vi "Main_SelectROI_on_ExtDispl.vi"() -> ()   [LabVIEW 2020]
panel:
  out "ROI Descriptor":T1 {"Contours"."Type" items=["No Selection", "Point", "Line", "Rectangle", "Oval", "Polygon", "Freehand Region", "Annulus", "Unused2", "Unused3", "Broken Line", "Freehand Line", "Rotated Rectangle"]}
  in  "Event Button":bool
  out "Image":T2(plugin-control)
  out "error OUT":errorcluster
  in  "stop":bool
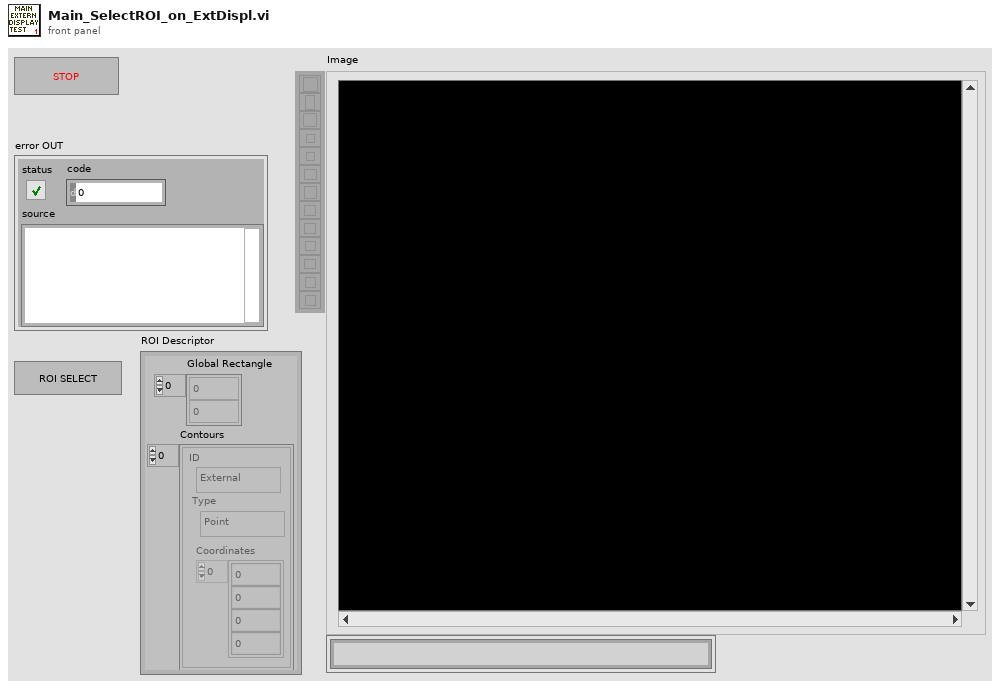
[diagram p1: front panel]
types:
  T1 = typedef "ROI Descriptor" = cluster{"Global Rectangle":i32[], "Contours":cluster{"ID":enum32{"External", "Internal"}, "Type":u32, "Coordinates":i32[]}[]}
  T2 = typedef "IMAQ Image.ctl" = refnum<image>
  T3 = typedef "Image Type" = u32
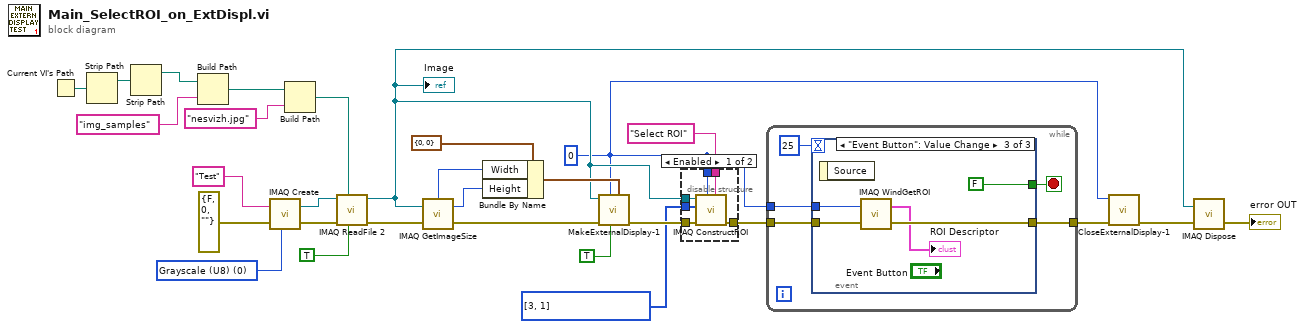
[diagram p0: block diagram]
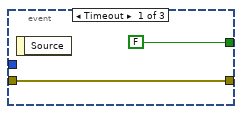
[diagram p3: hidden frame]
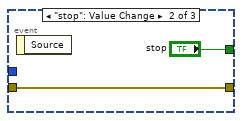
[diagram p4: hidden frame]
diagram:
  w9 = u32[] [3, 1] items=["No Selection", "Point", "Line", "Rectangle", "Oval", "Polygon", "Freehand Region", "Annulus", "Zoom", "Pan", "Broken Line", "Freehand Line", "Rotated Rectangle"] ("Tools")
  w8 = 0
  w27 = T3 0 items=["Grayscale (U8)", "Grayscale (I16)", "Grayscale (SGL)", "Complex (CSG)", "RGB (U32)", "HSL (U32)", "RGB (U64)", "Grayscale (U16)"] ("Image Type")
  n1 = Current VI's Path() -> (path=w4:path)
  n2 = Strip Path(path=w4) -> (stripped path=w3:path)  [unwired: 1 out]
  n3 = Strip Path(path=w3) -> (stripped path=w2:path)  [unwired: 1 out]
  n4 = Build Path(base path=w2, name or relative path="img_samples") -> (appended path=w5:path)
  n5 = call "IMAQ Create"("Image Name"="Test", "Image Type"=w27, "error in (no error)"=errorcluster {"status"=FALSE, "code"=0, "source"=""}) -> ("New Image"=w25:T2, "error out"=w26:errorcluster)  [unwired: 2 in]
  n6 = Build Path(base path=w5, name or relative path="nesvizh.jpg") -> (appended path=w1:path)
  n7 = call "IMAQ ReadFile 2"("Use File Path Image Type"=TRUE, "File Path"=w1, "error in (no error)"=w26, "Image"=w25) -> ("error out"=w21:errorcluster, "Image Out"=w11:T2)  [unwired: 3 in, 3 out]
  "Image" <- w11
  n8 = call "IMAQ GetImageSize"("Image"=w11, "error in (no error)"=w21) -> ("Y Resolution"=w18:i32, "X Resolution"=w19:i32, "error out"=w16:errorcluster)  [unwired: 2 in]
  n9 = Bundle By Name(cluster=cluster{"Width":i32, "Height":i32} {"Width"=0, "Height"=0} ("[IN] WxH"), "Width"=w19, "Height"=w18) -> (w17:cluster{"Width":i32, "Height":i32})
  n10 = call "MakeExternalDisplay-1.vi"("[IN] WxH"=w17, "[IN] Resize to Img Size?"=TRUE, "[IN] # Window"=w8, "error IN"=w16, "[IN] Image"=w11) -> ("error OUT"=w13:errorcluster)  [unwired: 6 in]
  n11 = disable-structure shown="Enabled" {
    disable-tunnel: w13 -> [w35 w36]
    disable-tunnel: [w34 w36] -> w12
    disable-tunnel: w11 -> [w33 _]
    disable-tunnel: "Select ROI" ("Prompt") -> [w32 _]
    disable-tunnel: w9 -> [w31 _]
    disable-tunnel: w8 -> [w30 _]
    frame Enabled {
      n12 = call "IMAQ ConstructROI"("Prompt"=w32, "Window Number (-1...15)"=w30, "error in (no error)"=w35, "Tools"=w31, "Image"=w33) -> ("error out"=w34:errorcluster)  [unwired: 3 in, 3 out]
    }
    frame Disabled {
    }
  }
  n13 = while {
    tunnel: w12 -> [w39]
    tunnel: [w38] -> w15
    tunnel: w8 -> [w37]
    stop <- w41 stop-if-true
    n14 = event shown="[2] \"Event Button\": Value Change" {
      selector: _ -> [_ _ _]
      dyn-events: _ -> [_ _ _]
      timeout: 25 -> [_ _ _]
      tunnel: [FALSE ("stop") "stop" FALSE ("stop")] -> w41
      tunnel: w39 -> [w42 w44 w49]
      tunnel: [w42 w44 w47] -> w38
      tunnel: w37 -> [_ _ w48]
      event Timeout {
        n15 = event-data() -> ()  [unwired: 1 in, 1 out]
      }
      event "stop": Value Change {
        n16 = event-data() -> ()  [unwired: 1 in, 1 out]
      }
      event "Event Button": Value Change {
        n17 = event-data() -> ()  [unwired: 1 in, 1 out]
        n18 = call "IMAQ WindGetROI"("Window Number (0...15)"=w48, "error in (no error)"=w49) -> ("ROI Descriptor"=→"ROI Descriptor":T1, "error out"=w47:errorcluster)  [unwired: 3 in]
      }
    }
  }
  n19 = call "CloseExternalDisplay-1.vi"("error IN"=w15, "[IN] # Window"=w8) -> ("error OUT"=w14:errorcluster)  [unwired: 5 in]
  n20 = call "IMAQ Dispose"("Image"=w11, "error in (no error)"=w14) -> ("error out"=→"error OUT":errorcluster)  [unwired: 4 in]
